vi "GetProbePlanCoordinates.vi"(8 "Use index as X coord":bool=TRUE, 9 "Probe Card Channels":i32=1) -> (0 "file path":string, 2 "OK?":bool, 3 "Array":T1(array[cluster]))   [LabVIEW 2018] (continued)
961\tX=-194.39\ty=30873.63 \nLabel=Strip\t962\tX=147.77\ty=30983.95 \nLabel=Strip\t963\tX=-206.37\ty=31022.23 \nLabel=Strip\t964\tX=135.75\ty=31132.68 \nLabel=Strip\t965\tX=-218.40\ty=31170.82 \nLabel=Strip\t966\tX=123.67\ty=31281.41 \nLabel=Strip\t967\tX=-230.49\ty=31319.41 \nLabel=Strip\t968\tX=111.54\ty=31430.13 \nLabel=Strip\t969\tX=-242.64\ty=31468.00 \nLabel=Strip\t970\tX=99.34\ty=31578.85 \nLabel=Strip\t971\tX=-254.85\ty=31616.58 \nLabel=Strip\t972\tX=87.09\ty=31727.56 \nLabel=Strip\t973\tX=-267.12\ty=31765.16 \nLabel=Strip\t974\tX=74.79\ty=31876.28 \nLabel=Strip\t975\tX=-279.44\ty=31913.74 \nLabel=Strip\t976\tX=62.42\ty=32024.98 \nLabel=Strip\t977\tX=-291.82\ty=32062.31 \nLabel=Strip\t978\tX=49.99\ty=32173.69 \nLabel=Strip\t979\tX=-304.26\ty=32210.88 \nLabel=Strip\t980\tX=37.51\ty=32322.39 \nLabel=Strip\t981\tX=-316.76\ty=32359.44 \nLabel=Strip\t982\tX=24.97\ty=32471.09 \nLabel=Strip\t983\tX=-329.31\ty=32508.01 \nLabel=Strip\t984\tX=12.38\ty=32619.78 \nLabel=Strip\t985\tX=-341.92\ty=32656.56 \nLabel=Strip\t986\tX=-0.28\ty=32768.47 \nLabel=Strip\t987\tX=-354.59\ty=32805.12 \nLabel=Strip\t988\tX=-12.99\ty=32917.16 \nLabel=Strip\t989\tX=-367.32\ty=32953.67 \nLabel=Strip\t990\tX=-25.76\ty=33065.85 \nLabel=Strip\t991\tX=-380.10\ty=33102.22 \nLabel=Strip\t992\tX=-38.59\ty=33214.53 \nLabel=Strip\t993\tX=-392.94\ty=33250.76 \nLabel=Strip\t994\tX=-51.47\ty=33363.20 \nLabel=Strip\t995\tX=-405.84\ty=33399.30 \nLabel=Strip\t996\tX=-64.41\ty=33511.88 \nLabel=Strip\t997\tX=-418.80\ty=33547.84 \nLabel=Strip\t998\tX=-77.42\ty=33660.55 \nLabel=Strip\t999\tX=-431.81\ty=33696.37 \nLabel=Strip\t1000\tX=-90.47\ty=33809.21 \nLabel=Strip\t1001\tX=-444.88\ty=33844.90 \nLabel=Strip\t1002\tX=-103.59\ty=33957.87 \nLabel=Strip\t1003\tX=-458.01\ty=33993.43 \nLabel=Strip\t1004\tX=-116.76\ty=34106.53 \nLabel=Strip\t1005\tX=-471.20\ty=34141.95 \nLabel=Strip\t1006\tX=-129.99\ty=34255.18 \nLabel=Strip\t1007\tX=-484.45\ty=34290.47 \nLabel=Strip\t1008\tX=-143.28\ty=34403.83 \nLabel=Strip\t1009\tX=-497.75\ty=34438.98 \nLabel=Strip\t1010\tX=-156.63\ty=34552.48 \nLabel=Strip\t1011\tX=-511.11\ty=34587.49 \nLabel=Strip\t1012\tX=-170.03\ty=34701.12 \nLabel=Strip\t1013\tX=-524.53\ty=34736.00 \nLabel=Strip\t1014\tX=-183.49\ty=34849.76 \nLabel=Strip\t1015\tX=-538.00\ty=34884.50 \nLabel=Strip\t1016\tX=-197.01\ty=34998.40 \nLabel=Strip\t1017\tX=-551.53\ty=35033.00 \nLabel=Strip\t1018\tX=-210.59\ty=35147.03 \nLabel=Strip\t1019\tX=-565.13\ty=35181.49 \nLabel=Strip\t1020\tX=-224.23\ty=35295.65 \nLabel=Strip\t1021\tX=-578.77\ty=35329.98 \nLabel=Strip\t1022\tX=-237.92\ty=35444.28 \nLabel=Strip\t1023\tX=-592.48\ty=35478.47 \nLabel=Strip\t1024\tX=-251.67\ty=35592.89 \nLabel=Strip\t1025\tX=-606.24\ty=35626.95 \nLabel=Strip\t1026\tX=-265.48\ty=35741.51 \nRegion=Segment\t3B\nLabel=Strip\t1\tX=16353.25\ty=-41866.46 \nLabel=Strip\t2\tX=16710.13\ty=-41818.03 \nLabel=Strip\t3\tX=16369.36\ty=-41712.09 \nLabel=Strip\t4\tX=16726.22\ty=-41663.53 \nLabel=Strip\t5\tX=16385.40\ty=-41557.71 \nLabel=Strip\t6\tX=16742.24\ty=-41509.01 \nLabel=Strip\t7\tX=16401.39\ty=-41403.33 \nLabel=Strip\t8\tX=16758.21\ty=-41354.49 \nLabel=Strip\t9\tX=16417.32\ty=-41248.94 \nLabel=Strip\t10\tX=16774.12\ty=-41199.96 \nLabel=Strip\t11\tX=16433.19\ty=-41094.54 \nLabel=Strip\t12\tX=16789.97\ty=-41045.43 \nLabel=Strip\t13\tX=16449.00\ty=-40940.14 \nLabel=Strip\t14\tX=16805.76\ty=-40890.88 \nLabel=Strip\t15\tX=16464.75\ty=-40785.73 \nLabel=Strip\t16\tX=16821.49\ty=-40736.33 \nLabel=Strip\t17\tX=16480.44\ty=-40631.31 \nLabel=Strip\t18\tX=16837.17\ty=-40581.78 \nLabel=Strip\t19\tX=16496.07\ty=-40476.88 \nLabel=Strip\t20\tX=16852.78\ty=-40427.21 \nLabel=Strip\t21\tX=16511.64\ty=-40322.44 \nLabel=Strip\t22\tX=16868.33\ty=-40272.64 \nLabel=Strip\t23\tX=16527.16\ty=-40168.00 \nLabel=Strip\t24\tX=16883.83\ty=-40118.06 \nLabel=Strip\t25\tX=16542.61\ty=-40013.55 \nLabel=Strip\t26\tX=16899.26\ty=-39963.47 \nLabel=Strip\t27\tX=16558.00\ty=-39859.10 \nLabel=Strip\t28\tX=16914.63\ty=-39808.88 \nLabel=Strip\t29\tX=16573.34\ty=-39704.63 \nLabel=Strip\t30\tX=16929.95\ty=-39654.27 \nLabel=Strip\t31\tX=16588.61\ty=-39550.16 \nLabel=Strip\t32\tX=16945.20\ty=-39499.66 \nLabel=Strip\t33\tX=16603.83\ty=-39395.69 \nLabel=Strip\t34\tX=16960.40\ty=-39345.05 \nLabel=Strip\t35\tX=16618.98\ty=-39241.20 \nLabel=Strip\t36\tX=16975.54\ty=-39190.43 \nLabel=Strip\t37\tX=16634.08\ty=-39086.71 \nLabel=Strip\t38\tX=16990.61\ty=-39035.80 \nLabel=Strip\t39\tX=16649.12\ty=-38932.21 \nLabel=Strip\t40\tX=17005.63\ty=-38881.16 \nLabel=Strip\t41\tX=16664.10\ty=-38777.70 \nLabel=Strip\t42\tX=17020.59\ty=-38726.51 \nLabel=Strip\t43\tX=16679.01\ty=-38623.19 \nLabel=Strip\t44\tX=17035.49\ty=-38571.86 \nLabel=Strip\t45\tX=16693.87\ty=-38468.67 \nLabel=Strip\t46\tX=17050.33\ty=-38417.20 \nLabel=Strip\t47\tX=16708.67\ty=-38314.14 \nLabel=Strip\t48\tX=17065.11\ty=-38262.54 \nLabel=Strip\t49\tX=16723.41\ty=-38159.61 \nLabel=Strip\t50\tX=17079.83\ty=-38107.86 \nLabel=Strip\t51\tX=16738.09\ty=-38005.07 \nLabel=Strip\t52\tX=17094.49\ty=-37953.18 \nLabel=Strip\t53\tX=16752.71\ty=-37850.52 \nLabel=Strip\t54\tX=17109.09\ty=-37798.50 \nLabel=Strip\t55\tX=16767.28\ty=-37695.96 \nLabel=Strip\t56\tX=17123.63\ty=-37643.80 \nLabel=Strip\t57\tX=16781.78\ty=-37541.40 \nLabel=Strip\t58\tX=17138.11\ty=-37489.10 \nLabel=Strip\t59\tX=16796.22\ty=-37386.83 \nLabel=Strip\t60\tX=17152.54\ty=-37334.40 \nLabel=Strip\t61\tX=16810.61\ty=-37232.26 \nLabel=Strip\t62\tX=17166.90\ty=-37179.68 \nLabel=Strip\t63\tX=16824.93\ty=-37077.67 \nLabel=Strip\t64\tX=17181.20\ty=-37024.96 \nLabel=Strip\t65\tX=16839.19\ty=-36923.08 \nLabel=Strip\t66\tX=17195.45\ty=-36870.23 \nLabel=Strip\t67\tX=16853.40\ty=-36768.49 \nLabel=Strip\t68\tX=17209.63\ty=-36715.50 \nLabel=Strip\t69\tX=16867.54\ty=-36613.89 \nLabel=Strip\t70\tX=17223.76\ty=-36560.76 \nLabel=Strip\t71\tX=16881.63\ty=-36459.28 \nLabel=Strip\t72\tX=17237.82\ty=-36406.01 \nLabel=Strip\t73\tX=16895.66\ty=-36304.66 \nLabel=Strip\t74\tX=17251.83\ty=-36251.26 \nLabel=Strip\t75\tX=16909.62\ty=-36150.04 \nLabel=Strip\t76\tX=17265.78\ty=-36096.49 \nLabel=Strip\t77\tX=16923.53\ty=-35995.41 \nLabel=Strip\t78\tX=17279.66\ty=-35941.73 \nLabel=Strip\t79\tX=16937.38\ty=-35840.77 \nLabel=Strip\t80\tX=17293.49\ty=-35786.95 \nLabel=Strip\t81\tX=16951.17\ty=-35686.13 \nLabel=Strip\t82\tX=17307.26\ty=-35632.17 \nLabel=Strip\t83\tX=16964.90\ty=-35531.48 \nLabel=Strip\t84\tX=17320.97\ty=-35477.38 \nLabel=Strip\t85\tX=16978.57\ty=-35376.82 \nLabel=Strip\t86\tX=17334.62\ty=-35322.59 \nLabel=Strip\t87\tX=16992.18\ty=-35222.16 \nLabel=Strip\t88\tX=17348.20\ty=-35167.79 \nLabel=Strip\t89\tX=17005.73\ty=-35067.49 \nLabel=Strip\t90\tX=17361.73\ty=-35012.98 \nLabel=Strip\t91\tX=17019.22\ty=-34912.81 \nLabel=Strip\t92\tX=17375.20\ty=-34858.17 \nLabel=Strip\t93\tX=17032.65\ty=-34758.13 \nLabel=Strip\t94\tX=17388.61\ty=-34703.35 \nLabel=Strip\t95\tX=17046.02\ty=-34603.44 \nLabel=Strip\t96\tX=17401.96\ty=-34548.52 \nLabel=Strip\t97\tX=17059.33\ty=-34448.75 \nLabel=Strip\t98\tX=17415.26\ty=-34393.68 \nLabel=Strip\t99\tX=17072.59\ty=-34294.04 \nLabel=Strip\t100\tX=17428.49\ty=-34238.85 \nLabel=Strip\t101\tX=17085.78\ty=-34139.34 \nLabel=Strip\t102\tX=17441.66\ty=-34084.00 \nLabel=Strip\t103\tX=17098.91\ty=-33984.62 \nLabel=Strip\t104\tX=17454.77\ty=-33929.15 \nLabel=Strip\t105\tX=17111.99\ty=-33829.90 \nLabel=Strip\t106\tX=17467.82\ty=-33774.29 \nLabel=Strip\t107\tX=17125.00\ty=-33675.17 \nLabel=Strip\t108\tX=17480.82\ty=-33619.42 \nLabel=Strip\t109\tX=17137.96\ty=-33520.44 \nLabel=Strip\t110\tX=17493.75\ty=-33464.55 \nLabel=Strip\t111\tX=17150.85\ty=-33365.70 \nLabel=Strip\t112\tX=17506.62\ty=-33309.67 \nLabel=Strip\t113\tX=17163.69\ty=-33210.95 \nLabel=Strip\t114\tX=17519.44\ty=-33154.79 \nLabel=Strip\t115\tX=17176.46\ty=-33056.20 \nLabel=Strip\t116\tX=17532.19\ty=-32999.90 \nLabel=Strip\t117\tX=17189.18\ty=-32901.44 \nLabel=Strip\t118\tX=17544.89\ty=-32845.00 \nLabel=Strip\t119\tX=17201.84\ty=-32746.68 \nLabel=Strip\t120\tX=17557.53\ty=-32690.10 \nLabel=Strip\t121\tX=17214.44\ty=-32591.91 \nLabel=Strip\t122\tX=17570.10\ty=-32535.19 \nLabel=Strip\t123\tX=17226.97\ty=-32437.13 \nLabel=Strip\t124\tX=17582.62\ty=-32380.28 \nLabel=Strip\t125\tX=17239.45\ty=-32282.35 \nLabel=Strip\t126\tX=17595.07\ty=-32225.35 \nLabel=Strip\t127\tX=17251.87\ty=-32127.65 \nLabel=Strip\t128\tX=17607.47\ty=-32070.43 \nLabel=Strip\t129\tX=17264.23\ty=-31972.76 \nLabel=Strip\t130\tX=17619.81\ty=-31915.49 \nLabel=Strip\t131\tX=17276.53\ty=-31817.96 \nLabel=Strip\t132\tX=17632.09\ty=-31760.55 \nLabel=Strip\t133\tX=17288.77\ty=-31663.15 \nLabel=Strip\t134\tX=17644.30\ty=-31605.61 \nLabel=Strip\t135\tX=17300.95\ty=-31508.34 \nLabel=Strip\t136\tX=17656.46\ty=-31450.66 \nLabel=Strip\t137\tX=17313.07\ty=-31353.52 \nLabel=Strip\t138\tX=17668.56\ty=-31295.70 \nLabel=Strip\t139\tX=17325.13\ty=-31198.70 \nLabel=Strip\t140\tX=17680.60\ty=-31140.74 \nLabel=Strip\t141\tX=17337.13\ty=-31043.86 \nLabel=Strip\t142\tX=17692.58\ty=-30985.77 \nLabel=Strip\t143\tX=17349.08\ty=-30889.03 \nLabel=Strip\t144\tX=17704.50\ty=-30830.79 \nLabel=Strip\t145\tX=17360.96\ty=-30734.18 \nLabel=Strip\t146\tX=17716.36\ty=-30675.81 \nLabel=Strip\t147\tX=17372.78\ty=-30579.33 \nLabel=Strip\t148\tX=17728.16\ty=-30520.82 \nLabel=Strip\t149\tX=17384.55\ty=-30424.48 \nLabel=Strip\t150\tX=17739.90\ty=-30365.83 \nLabel=Strip\t151\tX=17396.25\ty=-30269.62 \nLabel=Strip\t152\tX=17751.58\ty=-30210.83 \nLabel=Strip\t153\tX=17407.89\ty=-30114.75 \nLabel=Strip\t154\tX=17763.20\ty=-30055.83 \nLabel=Strip\t155\tX=17419.48\ty=-29959.88 \nLabel=Strip\t156\tX=17774.76\ty=-29900.82 \nLabel=Strip\t157\tX=17431.00\ty=-29805.00 \nLabel=Strip\t158\tX=17786.27\ty=-29745.80 \nLabel=Strip\t159\tX=17442.47\ty=-29650.12 \nLabel=Strip\t160\tX=17797.71\ty=-29590.78 \nLabel=Strip\t161\tX=17453.87\ty=-29495.23 \nLabel=Strip\t162\tX=17809.09\ty=-29435.75 \nLabel=Strip\t163\tX=17465.22\ty=-29340.33 \nLabel=Strip\t164\tX=17820.42\ty=-29280.72 \nLabel=Strip\t165\tX=17476.51\ty=-29185.43 \nLabel=Strip\t166\tX=17831.68\ty=-29125.68 \nLabel=Strip\t167\tX=17487.73\ty=-29030.53 \nLabel=Strip\t168\tX=17842.88\ty=-28970.64 \nLabel=Strip\t169\tX=17498.90\ty=-28875.61 \nLabel=Strip\t170\tX=17854.03\ty=-28815.59 \nLabel=Strip\t171\tX=17510.01\ty=-28720.70 \nLabel=Strip\t172\tX=17865.11\ty=-28660.53 \nLabel=Strip\t173\tX=17521.05\ty=-28565.77 \nLabel=Strip\t174\tX=17876.13\ty=-28505.47 \nLabel=Strip\t175\tX=17532.04\ty=-28410.84 \nLabel=Strip\t176\tX=17887.10\ty=-28350.41 \nLabel=Strip\t177\tX=17542.97\ty=-28255.91 \nLabel=Strip\t178\tX=17898.00\ty=-28195.33 \nLabel=Strip\t179\tX=17553.84\ty=-28100.97 \nLabel=Strip\t180\tX=17908.85\ty=-28040.25 \nLabel=Strip\t181\tX=17564.65\ty=-27946.03 \nLabel=Strip\t182\tX=17919.64\ty=-27885.17 \nLabel=Strip\t183\tX=17575.40\ty=-27791.07 \nLabel=Strip\t184\tX=17930.36\ty=-27730.08 \nLabel=Strip\t185\tX=17586.09\ty=-27636.12 \nLabel=Strip\t186\tX=17941.03\ty=-27574.99 \nLabel=Strip\t187\tX=17596.72\ty=-27481.16 \nLabel=Strip\t188\tX=17951.63\ty=-27419.89 \nLabel=Strip\t189\tX=17607.29\ty=-27326.19 \nLabel=Strip\t190\tX=17962.18\ty=-27264.79 \nLabel=Strip\t191\tX=17617.80\ty=-27171.22 \nLabel=Strip\t192\tX=17972.67\ty=-27109.68 \nLabel=Strip\t193\tX=17628.25\ty=-27016.24 \nLabel=Strip\t194\tX=17983.09\ty=-26954.56 \nLabel=Strip\t195\tX=17638.64\ty=-26861.26 \nLabel=Strip\t196\tX=17993.46\ty=-26799.44 \nLabel=Strip\t197\tX=17648.97\ty=-26706.27 \nLabel=Strip\t198\tX=18003.77\ty=-26644.31 \nLabel=Strip\t199\tX=17659.24\ty=-26551.27 \nLabel=Strip\t200\tX=18014.02\ty=-26489.18 \nLabel=Strip\t201\tX=17669.45\ty=-26396.28 \nLabel=Strip\t202\tX=18024.20\ty=-26334.05 \nLabel=Strip\t203\tX=17679.61\ty=-26241.27 \nLabel=Strip\t204\tX=18034.33\ty=-26178.90 \nLabel=Strip\t205\tX=17689.70\ty=-26086.26 \nLabel=Strip\t206\tX=18044.40\ty=-26023.76 \nLabel=Strip\t207\tX=17699.73\ty=-25931.25 \nLabel=Strip\t208\tX=18054.41\ty=-25868.60 \nLabel=Strip\t209\tX=17709.71\ty=-25776.23 \nLabel=Strip\t210\tX=18064.36\ty=-25713.45 \nLabel=Strip\t211\tX=17719.62\ty=-25621.20 \nLabel=Strip\t212\tX=18074.25\ty=-25558.28 \nLabel=Strip\t213\tX=17729.47\ty=-25466.17 \nLabel=Strip\t214\tX=18084.08\ty=-25403.12 \nLabel=Strip\t215\tX=17739.27\ty=-25311.14 \nLabel=Strip\t216\tX=18093.85\ty=-25247.94 \nLabel=Strip\t217\tX=17749.00\ty=-25156.10 \nLabel=Strip\t218\tX=18103.56\ty=-25092.77 \nLabel=Strip\t219\tX=17758.68\ty=-25001.05 \nLabel=Strip\t220\tX=18113.21\ty=-24937.58 \nLabel=Strip\t221\tX=17768.29\ty=-24846.00 \nLabel=Strip\t222\tX=18122.80\ty=-24782.40 \nLabel=Strip\t223\tX=17777.85\ty=-24690.95 \nLabel=Strip\t224\tX=18132.33\ty=-24627.20 \nLabel=Strip\t225\tX=17787.34\ty=-24535.89 \nLabel=Strip\t226\tX=18141.80\ty=-24472.01 \nLabel=Strip\t227\tX=17796.78\ty=-24380.82 \nLabel=Strip\t228\tX=18151.21\ty=-24316.80 \nLabel=Strip\t229\tX=17806.15\ty=-24225.75 \nLabel=Strip\t230\tX=18160.56\ty=-24161.59 \nLabel=Strip\t231\tX=17815.47\ty=-24070.68 \nLabel=Strip\t232\tX=18169.85\ty=-24006.38 \nLabel=Strip\t233\tX=17824.73\ty=-23915.60 \nLabel=Strip\t234\tX=18179.09\ty=-23851.17 \nLabel=Strip\t235\tX=17833.92\ty=-23760.51 \nLabel=Strip\t236\tX=18188.26\ty=-23695.94 \nLabel=Strip\t237\tX=17843.06\ty=-23605.42 \nLabel=Strip\t238\tX=18197.37\ty=-23540.72 \nLabel=Strip\t239\tX=17852.14\ty=-23450.33 \nLabel=Strip\t240\tX=18206.42\ty=-23385.48 \nLabel=Strip\t241\tX=17861.15\ty=-23295.23 \nLabel=Strip\t242\tX=18215.41\ty=-23230.25 \nLabel=Strip\t243\tX=17870.11\ty=-23140.12 \nLabel=Strip\t244\tX=18224.35\ty=-23075.01 \nLabel=Strip\t245\tX=17879.01\ty=-22985.02 \nLabel=Strip\t246\tX=18233.22\ty=-22919.76 \nLabel=Strip\t247\tX=17887.85\ty=-22829.90 \nLabel=Strip\t248\tX=18242.05\ty=-22764.05 \nLabel=Strip\t249\tX=17896.63\ty=-22674.78 \nLabel=Strip\t250\tX=18250.79\ty=-22609.25 \nLabel=Strip\t251\tX=17905.34\ty=-22519.66 \nLabel=Strip\t252\tX=18259.48\ty=-22453.99 \nLabel=Strip\t253\tX=17914.00\ty=-22364.53 \nLabel=Strip\t254\tX=18268.11\ty=-22298.73 \nLabel=Strip\t255\tX=17922.60\ty=-22209.40 \nLabel=Strip\t256\tX=18276.69\ty=-22143.46 \nLabel=Strip\t257\tX=17931.14\ty=-22054.27 \nLabel=Strip\t258\tX=18285.20\ty=-21988.18 \nLabel=Strip\t259\tX=17939.62\ty=-21899.12 \nLabel=Strip\t260\tX=18293.65\ty=-21832.91 \nLabel=Strip\t261\tX=17948.04\ty=-21743.98 \nLabel=Strip\t262\tX=18302.05\ty=-21677.62 \nLabel=Strip\t263\tX=17956.40\ty=-21588.83 \nLabel=Strip\t264\tX=18310.38\ty=-21522.33 \nLabel=Strip\t265\tX=17964.70\ty=-21433.67 \nLabel=Strip\t266\tX=18318.66\ty=-21367.04 \nLabel=Strip\t267\tX=17972.94\ty=-21278.51 \nLabel=Strip\t268\tX=18326.87\ty=-21211.75 \nLabel=Strip\t269\tX=17981.12\ty=-21123.35 \nLabel=Strip\t270\tX=18335.03\ty=-21056.44 \nLabel=Strip\t271\tX=17989.24\ty=-20968.18 \nLabel=Strip\t272\tX=18343.12\ty=-20901.14 \nLabel=Strip\t273\tX=17997.30\ty=-20813.01 \nLabel=Strip\t274\tX=18351.16\ty=-20745.83 \nLabel=Strip\t275\tX=18005.30\ty=-20657.83 \nLabel=Strip\t276\tX=18359.13\ty=-20590.51 \nLabel=Strip\t277\tX=18013.24\ty=-20502.65 \nLabel=Strip\t278\tX=18367.05\ty=-20435.20 \nLabel=Strip\t279\tX=18021.13\ty=-20347.46 \nLabel=Strip\t280\tX=18374.90\ty=-20279.87 \nLabel=Strip\t281\tX=18028.95\ty=-20192.27 \nLabel=Strip\t282\tX=18382.70\ty=-20124.55 \nLabel=Strip\t283\tX=18036.71\ty=-20037.08 \nLabel=Strip\t284\tX=18390.43\ty=-19969.21 \nLabel=Strip\t285\tX=18044.41\ty=-19881.88 \nLabel=Strip\t286\tX=18398.11\ty=-19813.88 \nLabel=Strip\t287\tX=18052.05\ty=-19726.68 \nLabel=Strip\t288\tX=18405.72\ty=-19658.54 \nLabel=Strip\t289\tX=18059.64\ty=-19571.47 \nLabel=Strip\t290\tX=18413.28\ty=-19503.19 \nLabel=Strip\t291\tX=18067.16\ty=-19416.26 \nLabel=Strip\t292\tX=18420.78\ty=-19347.84 \nLabel=Strip\t293\tX=18074.62\ty=-19261.04 \nLabel=Strip\t294\tX=18428.21\ty=-19192.49 \nLabel=Strip\t295\tX=18082.02\ty=-19105.82 \nLabel=Strip\t296\tX=18435.59\ty=-19037.13 \nLabel=Strip\t297\tX=18089.37\ty=-18950.60 \nLabel=Strip\t298\tX=18442.91\ty=-18881.77 \nLabel=Strip\t299\tX=18096.65\ty=-18795.37 \nLabel=Strip\t300\tX=18450.16\ty=-18726.41 \nLabel=Strip\t301\tX=18103.87\ty=-18640.14 \nLabel=Strip\t302\tX=18457.36\ty=-18571.04 \nLabel=Strip\t303\tX=18111.04\ty=-18484.90 \nLabel=Strip\t304\tX=18464.50\ty=-18415.66 \nLabel=Strip\t305\tX=18118.14\ty=-18329.66 \nLabel=Strip\t306\tX=18471.57\ty=-18260.29 \nLabel=Strip\t307\tX=18125.18\ty=-18174.42 \nLabel=Strip\t308\tX=18478.59\ty=-18104.90 \nLabel=Strip\t309\tX=18132.17\ty=-18019.17 \nLabel=Strip\t310\tX=18485.55\ty=-17949.52 \nLabel=Strip\t311\tX=18139.09\ty=-17863.91 \nLabel=Strip\t312\tX=18492.44\ty=-17794.13 \nLabel=Strip\t313\tX=18145.96\ty=-17708.66 \nLabel=Strip\t314\tX=18499.28\ty=-17638.73 \nLabel=Strip\t315\tX=18152.76\ty=-17553.40 \nLabel=Strip\t316\tX=18506.06\ty=-17483.34 \nLabel=Strip\t317\tX=18159.50\ty=-17398.13 \nLabel=Strip\t318\tX=18512.78\ty=-17327.94 \nLabel=Strip\t319\tX=18166.19\ty=-17242.86 \nLabel=Strip\t320\tX=18519.43\ty=-17172.53 \nLabel=Strip\t321\tX=18172.81\ty=-17087.59 \nLabel=Strip\t322\tX=18526.03\ty=-17017.12 \nLabel=Strip\t323\tX=18179.38\ty=-16932.32 \nLabel=Strip\t324\tX=18532.57\ty=-16861.71 \nLabel=Strip\t325\tX=18185.88\ty=-16777.04 \nLabel=Strip\t326\tX=18539.05\ty=-16706.29 \nLabel=Strip\t327\tX=18192.33\ty=-16621.75 \nLabel=Strip\t328\tX=18545.46\ty=-16550.87 \nLabel=Strip\t329\tX=18198.71\ty=-16466.45 \nLabel=Strip\t330\tX=18551.82\ty=-16395.45 \nLabel=Strip\t331\tX=18205.04\ty=-16311.17 \nLabel=Strip\t332\tX=18558.12\ty=-16240.02 \nLabel=Strip\t333\tX=18211.30\ty=-16155.88 \nLabel=Strip\t334\tX=18564.36\ty=-16084.59 \nLabel=Strip\t335\tX=18217.51\ty=-16000.58 \nLabel=Strip\t336\tX=18570.54\ty=-15929.15 \nLabel=Strip\t337\tX=18223.66\ty=-15845.28 \nLabel=Strip\t338\tX=18576.65\ty=-15773.71 \nLabel=Strip\t339\tX=18229.74\ty=-15689.97 \nLabel=Strip\t340\tX=18582.71\ty=-15618.27 \nLabel=Strip\t341\tX=18235.77\ty=-15534.66 \nLabel=Strip\t342\tX=18588.71\ty=-15462.82 \nLabel=Strip\t343\tX=18241.73\ty=-15379.35 \nLabel=Strip\t344\tX=18594.65\ty=-15307.37 \nLabel=Strip\t345\tX=18247.64\ty=-15224.03 \nLabel=Strip\t346\tX=18600.53\ty=-15151.92 \nLabel=Strip\t347\tX=18253.49\ty=-15068.71 \nLabel=Strip\t348\tX=18606.35\ty=-14996.46 \nLabel=Strip\t349\tX=18259.27\ty=-14913.39 \nLabel=Strip\t350\tX=18612.10\ty=-14841.00 \nLabel=Strip\t351\tX=18265.00\ty=-14758.06 \nLabel=Strip\t352\tX=18617.80\ty=-14685.53 \nLabel=Strip\t353\tX=18270.67\ty=-14602.73 \nLabel=Strip\t354\tX=18623.44\ty=-14530.07 \nLabel=Strip\t355\tX=18276.27\ty=-14447.40 \nLabel=Strip\t356\tX=18629.02\ty=-14374.60 \nLabel=Strip\t357\tX=18281.82\ty=-14292.06 \nLabel=Strip\t358\tX=18634.54\ty=-14219.12 \nLabel=Strip\t359\tX=18287.31\ty=-14136.72 \nLabel=Strip\t360\tX=18640.00\ty=-14063.64 \nLabel=Strip\t361\tX=18292.73\ty=-13981.37 \nLabel=Strip\t362\tX=18645.40\ty=-13908.16 \nLabel=Strip\t363\tX=18298.10\ty=-13826.02 \nLabel=Strip\t364\tX=18650.73\ty=-13752.68 \nLabel=Strip\t365\tX=18303.41\ty=-13670.67 \nLabel=Strip\t366\tX=18656.01\ty=-13597.19 \nLabel=Strip\t367\tX=18308.65\ty=-13515.32 \nLabel=Strip\t368\tX=18661.23\ty=-13441.70 \nLabel=Strip\t369\tX=18313.84\ty=-13359.96 \nLabel=Strip\t370\tX=18666.39\ty=-13286.20 \nLabel=Strip\t371\tX=18318.97\ty=-13204.60 \nLabel=Strip\t372\tX=18671.49\ty=-13130.70 \nLabel=Strip\t373\tX=18324.04\ty=-13049.23 \nLabel=Strip\t374\tX=18676.53\ty=-12975.20 \nLabel=Strip\t375\tX=18329.04\ty=-12893.86 \nLabel=Strip\t376\tX=18681.51\ty=-12819.70 \nLabel=Strip\t377\tX=18333.99\ty=-12738.49 \nLabel=Strip\t378\tX=18686.43\ty=-12664.19 \nLabel=Strip\t379\tX=18338.88\ty=-12583.12 \nLabel=Strip\t380\tX=18691.28\ty=-12508.68 \nLabel=Strip\t381\tX=18343.71\ty=-12427.74 \nLabel=Strip\t382\tX=18696.08\ty=-12353.16 \nLabel=Strip\t383\tX=18348.47\ty=-12272.36 \nLabel=Strip\t384\tX=18700.82\ty=-12197.64 \nLabel=Strip\t385\tX=18353.18\ty=-12116.98 \nLabel=Strip\t386\tX=18705.50\ty=-12042.12 \nLabel=Strip\t387\tX=18357.83\ty=-11961.59 \nLabel=Strip\t388\tX=18710.12\ty=-11886.60 \nLabel=Strip\t389\tX=18362.42\ty=-11806.20 \nLabel=Strip\t390\tX=18714.68\ty=-11731.07 \nLabel=Strip\t391\tX=18366.94\ty=-11650.80 \nLabel=Strip\t392\tX=18719.18\ty=-11575.54 \nLabel=Strip\t393\tX=18371.41\ty=-11495.41 \nLabel=Strip\t394\tX=18723.62\ty=-11420.01 \nLabel=Strip\t395\tX=18375.82\ty=-11340.01 \nLabel=Strip\t396\tX=18728.00\ty=-11264.47 \nLabel=Strip\t397\tX=18380.17\ty=-11184.61 \nLabel=Strip\t398\tX=18732.31\ty=-11108.93 \nLabel=Strip\t399\tX=18384.46\ty=-11029.20 \nLabel=Strip\t400\tX=18736.57\ty=-10953.39 \nLabel=Strip\t401\tX=18388.68\ty=-10873.79 \nLabel=Strip\t402\tX=18740.77\ty=-10797.85 \nLabel=Strip\t403\tX=18392.85\ty=-10718.38 \nLabel=Strip\t404\tX=18744.91\ty=-10642.30 \nLabel=Strip\t405\tX=18397.03\ty=-10545.69 \nLabel=Strip\t406\tX=18749.04\ty=-10472.72 \nLabel=Strip\t407\tX=18401.05\ty=-10397.30 \nLabel=Strip\t408\tX=18753.03\ty=-10324.33 \nLabel=Strip\t409\tX=18405.01\ty=-10248.90 \nLabel=Strip\t410\tX=18756.97\ty=-10175.93 \nLabel=Strip\t411\tX=18408.91\ty=-10100.50 \nLabel=Strip\t412\tX=18760.84\ty=-10027.53 \nLabel=Strip\t413\tX=18412.76\ty=-9952.10 \nLabel=Strip\t414\tX=18764.66\ty=-9879.13 \nLabel=Strip\t415\tX=18416.55\ty=-9803.70 \nLabel=Strip\t416\tX=18768.48\ty=-9708.95 \nLabel=Strip\t417\tX=18420.35\ty=-9630.42 \nLabel=Strip\t418\tX=18772.20\ty=-9553.39 \nLabel=Strip\t419\tX=18424.04\ty=-9474.99 \nLabel=Strip\t420\tX=18775.86\ty=-9397.82 \nLabel=Strip\t421\tX=18427.67\ty=-9319.55 \nLabel=Strip\t422\tX=18779.46\ty=-9242.24 \nLabel=Strip\t423\tX=18431.23\ty=-9164.11 \nLabel=Strip\t424\tX=18783.00\ty=-9086.67 \nLabel=Strip\t425\tX=18434.74\ty=-9008.67 \nLabel=Strip\t426\tX=18786.48\ty=-8931.09 \nLabel=Strip\t427\tX=18438.19\ty=-8853.23 \nLabel=Strip\t428\tX=18789.89\ty=-8775.51 \nLabel=Strip\t429\tX=18441.58\ty=-8697.78 \nLabel=Strip\t430\tX=18793.25\ty=-8619.92 \nLabel=Strip\t431\tX=18444.91\ty=-8542.33 \nLabel=Strip\t432\tX=18796.55\ty=-8464.34 \nLabel=Strip\t433\tX=18448.18\ty=-8386.88 \nLabel=Strip\t434\tX=18799.79\ty=-8308.75 \nLabel=Strip\t435\tX=18451.39\ty=-8231.42 \nLabel=Strip\t436\tX=18802.97\ty=-8153.16 \nLabel=Strip\t437\tX=18454.53\ty=-8075.97 \nLabel=Strip\t438\tX=18806.08\ty=-7997.56 \nLabel=Strip\t439\tX=18457.62\ty=-7920.51 \nLabel=Strip\t440\tX=18809.14\ty=-7841.97 \nLabel=Strip\t441\tX=18460.65\ty=-7765.04 \nLabel=Strip\t442\tX=18812.14\ty=-7686.37 \nLabel=Strip\t443\tX=18463.62\ty=-7609.58 \nLabel=Strip\t444\tX=18815.08\ty=-7530.77 \nLabel=Strip\t445\tX=18466.53\ty=-7454.11 \nLabel=Strip\t446\tX=18817.96\ty=-7375.16 \nLabel=Strip\t447\tX=18469.38\ty=-7298.64 \nLabel=Strip\t448\tX=18820.77\ty=-7219.56 \nLabel=Strip\t449\tX=18472.16\ty=-7143.17 \nLabel=Strip\t450\tX=18823.53\ty=-7063.95 \nLabel=Strip\t451\tX=18474.89\ty=-6987.70 \nLabel=Strip\t452\tX=18826.23\ty=-6908.34 \nLabel=Strip\t453\tX=18477.56\ty=-6832.22 \nLabel=Strip\t454\tX=18828.87\ty=-6752.73 \nLabel=Strip\t455\tX=18480.17\ty=-6676.74 \nLabel=Strip\t456\tX=18831.45\ty=-6597.11 \nLabel=Strip\t457\tX=18482.72\ty=-6521.26 \nLabel=Strip\t458\tX=18833.96\ty=-6441.49 \nLabel=Strip\t459\tX=18485.21\ty=-6365.77 \nLabel=Strip\t460\tX=18836.42\ty=-6285.87 \nLabel=Strip\t461\tX=18487.63\ty=-6210.29 \nLabel=Strip\t462\tX=18838.82\ty=-6130.25 \nLabel=Strip\t463\tX=18490.00\ty=-6054.80 \nLabel=Strip\t464\tX=18841.16\ty=-5974.62 \nLabel=Strip\t465\tX=18492.31\ty=-5899.31 \nLabel=Strip\t466\tX=18843.43\ty=-5819.00 \nLabel=Strip\t467\tX=18494.56\ty=-5743.82 \nLabel=Strip\t468\tX=18845.65\ty=-5663.37 \nLabel=Strip\t469\tX=18496.75\ty=-5588.32 \nLabel=Strip\t470\tX=18847.81\ty=-5507.74 \nLabel=Strip\t471\tX=18498.88\ty=-5432.82 \nLabel=Strip\t472\tX=18849.90\ty=-5352.10 \nLabel=Strip\t473\tX=18500.94\ty=-5277.33 \nLabel=Strip\t474\tX=18851.94\ty=-5196.47 \nLabel=Strip\t475\tX=18502.95\ty=-5121.82 \nLabel=Strip\t476\tX=18853.92\ty=-5040.83 \nLabel=Strip\t477\tX=18504.90\ty=-4966.32 \nLabel=Strip\t478\tX=18855.83\ty=-4885.19 \nLabel=Strip\t479\tX=18506.79\ty=-4810.82 \nLabel=Strip\t480\tX=18857.69\ty=-4729.55 \nLabel=Strip\t481\tX=18508.62\ty=-4655.31 \nLabel=Strip\t482\tX=18859.49\ty=-4573.91 \nLabel=Strip\t483\tX=18510.38\ty=-4499.80 \nLabel=Strip\t484\tX=18861.22\ty=-4418.26 \nLabel=Strip\t485\tX=18512.09\ty=-4344.29 \nLabel=Strip\t486\tX=18862.90\ty=-4262.62 \nLabel=Strip\t487\tX=18513.74\ty=-4188.77 \nLabel=Strip\t488\tX=18864.52\ty=-4106.97 \nLabel=Strip\t489\tX=18515.33\ty=-4033.26 \nLabel=Strip\t490\tX=18866.07\ty=-3951.31 \nLabel=Strip\t491\tX=18516.85\ty=-3877.74 \nLabel=Strip\t492\tX=18867.57\ty=-3795.66 \nLabel=Strip\t493\tX=18518.32\ty=-3722.22 \nLabel=Strip\t494\tX=18869.00\ty=-3640.01 \nLabel=Strip\t495\tX=18519.73\ty=-3566.70 \nLabel=Strip\t496\tX=18870.38\ty=-3484.35 \nLabel=Strip\t497\tX=18521.08\ty=-3411.18 \nLabel=Strip\t498\tX=18871.70\ty=-3328.69 \nLabel=Strip\t499\tX=18522.37\ty=-3255.66 \nLabel=Strip\t500\tX=18872.95\ty=-3173.03 \nLabel=Strip\t501\tX=18523.59\ty=-3100.13 \nLabel=Strip\t502\tX=18874.15\ty=-3017.37 \nLabel=Strip\t503\tX=18524.76\ty=-2944.60 \nLabel=Strip\t504\tX=18875.28\ty=-2861.70 \nLabel=Strip\t505\tX=18525.87\ty=-2789.07 \nLabel=Strip\t506\tX=18876.36\ty=-2706.02 \nLabel=Strip\t507\tX=18526.91\ty=-2633.54 \nLabel=Strip\t508\tX=18877.37\ty=-2550.37 \nLabel=Strip\t509\tX=18527.90\ty=-2478.01 \nLabel=Strip\t510\tX=18878.33\ty=-2394.70 \nLabel=Strip\t511\tX=18528.83\ty=-2322.47 \nLabel=Strip\t512\tX=18879.22\ty=-2239.03 \nLabel=Strip\t513\tX=18529.70\ty=-2166.93 \nLabel=Strip\t514\tX=18880.06\ty=-2083.36 \nLabel=Strip\t515\tX=18530.50\ty=-2011.40 \nLabel=Strip\t516\tX=18880.83\ty=-1927.68 \nLabel=Strip\t517\tX=18531.25\ty=-1855.86 \nLabel=Strip\t518\tX=18881.55\ty=-1772.01 \nLabel=Strip\t519\tX=18531.94\ty=-1700.31 \nLabel=Strip\t520\tX=18882.20\ty=-1616.33 \nLabel=Strip\t521\tX=18532.56\ty=-1544.77 \nLabel=Strip\t522\tX=18882.80\ty=-1460.65 \nLabel=Strip\t523\tX=18533.13\ty=-1389.23 \nLabel=Strip\t524\tX=18883.33\ty=-1304.97 \nLabel=Strip\t525\tX=18533.64\ty=-1233.68 \nLabel=Strip\t526\tX=18883.81\ty=-1149.29 \nLabel=Strip\t527\tX=18534.08\ty=-1078.13 \nLabel=Strip\t528\tX=18884.22\ty=-993.61 \nLabel=Strip\t529\tX=18534.47\ty=-922.58 \nLabel=Strip\t530\tX=18884.57\ty=-837.92 \nLabel=Strip\t531\tX=18534.80\ty=-767.03 \nLabel=Strip\t532\tX=18884.87\ty=-682.23 \nLabel=Strip\t533\tX=18535.06\ty=-611.48 \nLabel=Strip\t534\tX=18885.10\ty=-526.55 \nLabel=Strip\t535\tX=18535.27\ty=-455.93 \nLabel=Strip\t536\tX=18885.27\ty=-370.86 \nLabel=Strip\t537\tX=18535.42\ty=-300.37 \nLabel=Strip\t538\tX=18885.39\ty=-215.17 \nLabel=Strip\t539\tX=18535.50\ty=-144.82 \nLabel=Strip\t540\tX=18885.44\ty=-59.47 \nLabel=Strip\t541\tX=18535.53\ty=10.74 \nLabel=Strip\t542\tX=18885.43\ty=96.22 \nLabel=Strip\t543\tX=18535.49\ty=166.30 \nLabel=Strip\t544\tX=18885.37\ty=251.91 \nLabel=Strip\t545\tX=18535.40\ty=321.86 \nLabel=Strip\t546\tX=18885.24\ty=407.61 \nLabel=Strip\t547\tX=18535.25\ty=477.42 \nLabel=Strip\t548\tX=18885.05\ty=563.31 \nLabel=Strip\t549\tX=18535.03\ty=632.98 \nLabel=Strip\t550\tX=18884.80\ty=719.00 \nLabel=Strip\t551\tX=18534.76\ty=788.54 \nLabel=Strip\t552\tX=18884.50\ty=874.70 \nLabel=Strip\t553\tX=18534.42\ty=944.11 \nLabel=Strip\t554\tX=18884.13\ty=1030.40 \nLabel=Strip\t555\tX=18534.03\ty=1099.68 \nLabel=Strip\t556\tX=18883.70\ty=1186.10 \nLabel=Strip\t557\tX=18533.57\ty=1255.24 \nLabel=Strip\t558\tX=18883.21\ty=1341.81 \nLabel=Strip\t559\tX=18533.06\ty=1410.81 \nLabel=Strip\t560\tX=18882.66\ty=1497.51 \nLabel=Strip\t561\tX=18532.48\ty=1566.38 \nLabel=Strip\t562\tX=18882.05\ty=1653.22 \nLabel=Strip\t563\tX=18531.85\ty=1721.95 \nLabel=Strip\t564\tX=18881.39\ty=1808.92 \nLabel=Strip\t565\tX=18531.15\ty=1877.52 \nLabel=Strip\t566\tX=18880.66\ty=1964.63 \nLabel=Strip\t567\tX=18530.40\ty=2033.09 \nLabel=Strip\t568\tX=18879.87\ty=2120.34 \nLabel=Strip\t569\tX=18529.58\ty=2188.67 \nLabel=Strip\t570\tX=18879.02\ty=2276.05 \nLabel=Strip\t571\tX=18528.71\ty=2344.24 \nLabel=Strip\t572\tX=18878.11\ty=2431.76 \nLabel=Strip\t573\tX=18527.77\ty=2499.82 \nLabel=Strip\t574\tX=18877.14\ty=2587.47 \nLabel=Strip\t575\tX=18526.77\ty=2655.39 \nLabel=Strip\t576\tX=18876.11\ty=2743.18 \nLabel=Strip\t577\tX=18525.72\ty=2810.97 \nLabel=Strip\t578\tX=18875.02\ty=2898.89 \nLabel=Strip\t579\tX=18524.60\ty=2966.55 \nLabel=Strip\t580\tX=18873.87\ty=3054.61 \nLabel=Strip\t581\tX=18523.43\ty=3122.13 \nLabel=Strip\t582\tX=18872.66\ty=3210.32 \nLabel=Strip\t583\tX=18522.19\ty=3277.71 \nLabel=Strip\t584\tX=18871.39\ty=3366.04 \nLabel=Strip\t585\tX=18520.89\ty=3433.29 \nLabel=Strip\t586\tX=18870.06\ty=3521.75 \nLabel=Strip\t587\tX=18519.54\ty=3588.87 \nLabel=Strip\t588\tX=18868.67\ty=3677.47 \nLabel=Strip\t589\tX=18518.12\ty=3744.45 \nLabel=Strip\t590\tX=18867.22\ty=3833.19 \nLabel=Strip\t591\tX=18516.64\ty=3900.04 \nLabel=Strip\t592\tX=18865.71\ty=3988.91 \nLabel=Strip\t593\tX=18515.11\ty=4055.62 \nLabel=Strip\t594\tX=18864.14\ty=4144.63 \nLabel=Strip\t595\tX=18513.51\ty=4211.20 \nLabel=Strip\t596\tX=18862.50\ty=4300.34 \nLabel=Strip\t597\tX=18511.85\ty=4366.79 \nLabel=Strip\t598\tX=18860.81\ty=4456.07 \nLabel=Strip\t599\tX=18510.14\ty=4522.38 \nLabel=Strip\t600\tX=18859.06\ty=4611.79 \nLabel=Strip\t601\tX=18508.36\ty=4677.96 \nLabel=Strip\t602\tX=18857.25\ty=4767.51 \nLabel=Strip\t603\tX=18506.52\ty=4833.55 \nLabel=Strip\t604\tX=18855.38\ty=4923.23 \nLabel=Strip\t605\tX=18504.62\ty=4989.14 \nLabel=Strip\t606\tX=18853.45\ty=5078.95 \nLabel=Strip\t607\tX=18502.67\ty=5144.73 \nLabel=Strip\t608\tX=18851.45\ty=5234.68 \nLabel=Strip\t609\tX=18500.65\ty=5300.31 \nLabel=Strip\t610\tX=18849.40\ty=5390.40 \nLabel=Strip\t611\tX=18498.57\ty=5455.90 \nLabel=Strip\t612\tX=18847.29\ty=5546.13 \nLabel=Strip\t613\tX=18496.43\ty=5611.49 \nLabel=Strip\t614\tX=18845.11\ty=5701.85 \nLabel=Strip\t615\tX=18494.23\ty=5767.08 \nLabel=Strip\t616\tX=18842.88\ty=5857.58 \nLabel=Strip\t617\tX=18491.97\ty=5922.67 \nLabel=Strip\t618\tX=18840.59\ty=6013.30 \nLabel=Strip\t619\tX=18489.66\ty=6078.26 \nLabel=Strip\t620\tX=18838.23\ty=6169.03 \nLabel=Strip\t621\tX=18487.28\ty=6233.86 \nLabel=Strip\t622\tX=18835.82\ty=6324.76 \nLabel=Strip\t623\tX=18484.84\ty=6389.45 \nLabel=Strip\t624\tX=18833.35\ty=6480.48 \nLabel=Strip\t625\tX=18482.34\ty=6545.04 \nLabel=Strip\t626\tX=18830.81\ty=6636.21 \nLabel=Strip\t627\tX=18479.78\ty=6700.63 \nLabel=Strip\t628\tX=18828.22\ty=6791.94 \nLabel=Strip\t629\tX=18477.16\ty=6856.23 \nLabel=Strip\t630\tX=18825.56\ty=6947.67 \nLabel=Strip\t631\tX=18474.48\ty=7011.82 \nLabel=Strip\t632\tX=18822.85\ty=7103.40 \nLabel=Strip\t633\tX=18471.74\ty=7167.41 \nLabel=Strip\t634\tX=18820.07\ty=7259.12 \nLabel=Strip\t635\tX=18468.94\ty=7323.01 \nLabel=Strip\t636\tX=18817.24\ty=7414.85 \nLabel=Strip\t637\tX=18466.08\ty=7478.60 \nLabel=Strip\t638\tX=18814.34\ty=7570.58 \nLabel=Strip\t639\tX=18463.16\ty=7634.19 \nLabel=Strip\t640\tX=18811.39\ty=7726.31 \nLabel=Strip\t641\tX=18460.18\ty=7789.79 \nLabel=Strip\t642\tX=18808.37\ty=7882.04 \nLabel=Strip\t643\tX=18457.14\ty=7945.38 \nLabel=Strip\t644\tX=18805.29\ty=8037.77 \nLabel=Strip\t645\tX=18454.04\ty=8100.98 \nLabel=Strip\t646\tX=18802.16\ty=8193.50 \nLabel=Strip\t647\tX=18450.88\ty=8256.57 \nLabel=Strip\t648\tX=18798.96\ty=8349.23 \nLabel=Strip\t649\tX=18447.66\ty=8412.17 \nLabel=Strip\t650\tX=18795.70\ty=8504.96 \nLabel=Strip\t651\tX=18444.38\ty=8567.76 \nLabel=Strip\t652\tX=18792.39\ty=8660.69 \nLabel=Strip\t653\tX=18441.04\ty=8723.36 \nLabel=Strip\t654\tX=18789.01\ty=8816.42 \nLabel=Strip\t655\tX=18437.64\ty=8878.95 \nLabel=Strip\t656\tX=18785.57\ty=8972.15 \nLabel=Strip\t657\tX=18434.17\ty=9034.54 \nLabel=Strip\t658\tX=18782.08\ty=9127.88 \nLabel=Strip\t659\tX=18430.65\ty=9190.14 \nLabel=Strip\t660\tX=18778.52\ty=9283.61 \nLabel=Strip\t661\tX=18427.07\ty=9345.73 \nLabel=Strip\t662\tX=18774.90\ty=9439.34 \nLabel=Strip\t663\tX=18423.43\ty=9501.33 \nLabel=Strip\t664\tX=18771.22\ty=9595.07 \nLabel=Strip\t665\tX=18419.73\ty=9656.92 \nLabel=Strip\t666\tX=18767.48\ty=9750.80 \nLabel=Strip\t667\tX=18415.96\ty=9812.52 \nLabel=Strip\t668\tX=18763.68\ty=9906.52 \nLabel=Strip\t669\tX=18412.14\ty=9968.11 \nLabel=Strip\t670\tX=18759.83\ty=10062.25 \nLabel=Strip\t671\tX=18408.26\ty=10123.71 \nLabel=Strip\t672\tX=18755.91\ty=10217.98 \nLabel=Strip\t673\tX=18404.32\ty=10279.30 \nLabel=Strip\t674\tX=18751.93\ty=10373.71 \nLabel=Strip\t675\tX=18400.31\ty=10434.89 \nLabel=Strip\t676\tX=18747.89\ty=10529.44 \nLabel=Strip\t677\tX=18396.25\ty=10590.49 \nLabel=Strip\t678\tX=18743.79\ty=10685.17 \nLabel=Strip\t679\tX=18392.13\ty=10746.08 \nLabel=Strip\t680\tX=18739.63\ty=10840.90 \nLabel=Strip\t681\tX=18387.94\ty=10901.67 \nLabel=Strip\t682\tX=18735.41\ty=10996.62 \nLabel=Strip\t683\tX=18383.70\ty=11057.26 \nLabel=Strip\t684\tX=18731.13\ty=11152.35 \nLabel=Strip\t685\tX=18379.40\ty=11212.86 \nLabel=Strip\t686\tX=18726.79\ty=11308.08 \nLabel=Strip\t687\tX=18375.03\ty=11368.45 \nLabel=Strip\t688\tX=18722.39\ty=11463.80 \nLabel=Strip\t689\tX=18370.61\ty=11524.04 \nLabel=Strip\t690\tX=18717.92\ty=11619.53 \nLabel=Strip\t691\tX=18366.12\ty=11679.63 \nLabel=Strip\t692\tX=18713.40\ty=11775.25 \nLabel=Strip\t693\tX=18361.58\ty=11835.22 \nLabel=Strip\t694\tX=18708.82\ty=11930.98 \nLabel=Strip\t695\tX=18356.97\ty=11990.81 \nLabel=Strip\t696\tX=18704.18\ty=12086.70 \nLabel=Strip\t697\tX=18352.31\ty=12146.40 \nLabel=Strip\t698\tX=18699.48\ty=12242.43 \nLabel=Strip\t699\tX=18347.58\ty=12301.99 \nLabel=Strip\t700\tX=18694.72\ty=12398.15 \nLabel=Strip\t701\tX=18342.80\ty=12457.58 \nLabel=Strip\t702\tX=18689.89\ty=12553.88 \nLabel=Strip\t703\tX=18337.95\ty=12613.16 \nLabel=Strip\t704\tX=18685.01\ty=12709.60 \nLabel=Strip\t705\tX=18333.05\ty=12768.75 \nLabel=Strip\t706\tX=18680.07\ty=12865.32 \nLabel=Strip\t707\tX=18328.08\ty=12924.34 \nLabel=Strip\t708\tX=18675.06\ty=13021.04 \nLabel=Strip\t709\tX=18323.05\ty=13079.92 \nLabel=Strip\t710\tX=18670.00\ty=13176.76 \nLabel=Strip\t711\tX=18317.97\ty=13235.51 \nLabel=Strip\t712\tX=18664.88\ty=13332.48 \nLabel=Strip\t713\tX=18312.82\ty=13391.09 \nLabel=Strip\t714\tX=18659.69\ty=13488.20 \nLabel=Strip\t715\tX=18307.62\ty=13546.68 \nLabel=Strip\t716\tX=18654.45\ty=13643.92 \nLabel=Strip\t717\tX=18302.35\ty=13702.26 \nLabel=Strip\t718\tX=18649.14\ty=13799.64 \nLabel=Strip\t719\tX=18297.02\ty=13857.84 \nLabel=Strip\t720\tX=18643.78\ty=13955.35 \nLabel=Strip\t721\tX=18291.63\ty=14013.43 \nLabel=Strip\t722\tX=18638.35\ty=14111.07 \nLabel=Strip\t723\tX=18286.19\ty=14169.01 \nLabel=Strip\t724\tX=18632.87\ty=14266.79 \nLabel=Strip\t725\tX=18280.68\ty=14324.59 \nLabel=Strip\t726\tX=18627.32\ty=14422.50 \nLabel=Strip\t727\tX=18275.11\ty=14480.17 \nLabel=Strip\t728\tX=18621.72\ty=14578.22 \nLabel=Strip\t729\tX=18269.48\ty=14635.75 \nLabel=Strip\t730\tX=18616.05\ty=14733.93 \nLabel=Strip\t731\tX=18263.80\ty=14791.32 \nLabel=Strip\t732\tX=18610.33\ty=14889.64 \nLabel=Strip\t733\tX=18258.01\ty=14947.56 \nLabel=Strip\t734\tX=18604.54\ty=15045.35 \nLabel=Strip\t735\tX=18252.24\ty=15102.47 \nLabel=Strip\t736\tX=18598.69\ty=15201.06 \nLabel=Strip\t737\tX=18246.37\ty=15258.05 \nLabel=Strip\t738\tX=18592.79\ty=15356.77 \nLabel=Strip\t739\tX=18240.44\ty=15413.62 \nLabel=Strip\t740\tX=18586.82\ty=15512.48 \nLabel=Strip\t741\tX=18234.45\ty=15569.20 \nLabel=Strip\t742\tX=18580.79\ty=15668.19 \nLabel=Strip\t743\tX=18228.40\ty=15724.77 \nLabel=Strip\t744\tX=18574.70\ty=15823.89 \nLabel=Strip\t745\tX=18222.29\ty=15880.34 \nLabel=Strip\t746\tX=18568.56\ty=15979.60 \nLabel=Strip\t747\tX=18216.12\ty=16035.91 \nLabel=Strip\t748\tX=18562.35\ty=16135.30 \nLabel=Strip\t749\tX=18209.89\ty=16191.48 \nLabel=Strip\t750\tX=18556.08\ty=16291.01 \nLabel=Strip\t751\tX=18203.60\ty=16347.05 \nLabel=Strip\t752\tX=18549.75\ty=16446.71 \nLabel=Strip\t753\tX=18197.25\ty=16502.61 \nLabel=Strip\t754\tX=18543.36\ty=16602.41 \nLabel=Strip\t755\tX=18190.84\ty=16658.18 \nLabel=Strip\t756\tX=18536.91\ty=16758.11 \nLabel=Strip\t757\tX=18184.37\ty=16813.74 \nLabel=Strip\t758\tX=18530.40\ty=16913.81 \nLabel=Strip\t759\tX=18177.84\ty=16969.30 \nLabel=Strip\t760\tX=18523.83\ty=17069.50 \nLabel=Strip\t761\tX=18171.25\ty=17124.87 \nLabel=Strip\t762\tX=18517.20\ty=17225.20 \nLabel=Strip\t763\tX=18164.60\ty=17280.43 \nLabel=Strip\t764\tX=18510.51\ty=17380.89 \nLabel=Strip\t765\tX=18157.89\ty=17435.99 \nLabel=Strip\t766\tX=18503.76\ty=17536.59 \nLabel=Strip\t767\tX=18151.11\ty=17591.54 \nLabel=Strip\t768\tX=18496.95\ty=17692.28 \nLabel=Strip\t769\tX=18144.28\ty=17747.10 \nLabel=Strip\t770\tX=18490.08\ty=17847.97 \nLabel=Strip\t771\tX=18137.39\ty=17902.65 \nLabel=Strip\t772\tX=18483.15\ty=18003.66 \nLabel=Strip\t773\tX=18130.44\ty=18058.21 \nLabel=Strip\t774\tX=18476.16\ty=18159.35 \nLabel=Strip\t775\tX=18123.43\ty=18213.76 \nLabel=Strip\t776\tX=18469.11\ty=18315.03 \nLabel=Strip\t777\tX=18116.35\ty=18369.31 \nLabel=Strip\t778\tX=18461.99\ty=18470.72 \nLabel=Strip\t779\tX=18109.22\ty=18524.86 \nLabel=Strip\t780\tX=18454.82\ty=18626.40 \nLabel=Strip\t781\tX=18102.03\ty=18680.41 \nLabel=Strip\t782\tX=18447.59\ty=18782.08 \nLabel=Strip\t783\tX=18094.77\ty=18835.96 \nLabel=Strip\t784\tX=18440.30\ty=18937.76 \nLabel=Strip\t785\tX=18087.46\ty=18991.50 \nLabel=Strip\t786\tX=18432.94\ty=19093.44 \nLabel=Strip\t787\tX=18080.09\ty=19147.04 \nLabel=Strip\t788\tX=18425.53\ty=19249.12 \nLabel=Strip\t789\tX=18072.65\ty=19302.59 \nLabel=Strip\t790\tX=18418.06\ty=19404.80 \nLabel=Strip\t791\tX=18065.16\ty=19458.13 \nLabel=Strip\t792\tX=18410.52\ty=19560.47 \nLabel=Strip\t793\tX=18057.60\ty=19613.66 \nLabel=Strip\t794\tX=18402.93\ty=19716.14 \nLabel=Strip\t795\tX=18049.99\ty=19769.20 \nLabel=Strip\t796\tX=18395.28\ty=19871.82 \nLabel=Strip\t797\tX=18042.31\ty=19924.74 \nLabel=Strip\t798\tX=18387.56\ty=20027.49 \nLabel=Strip\t799\tX=18034.58\ty=20080.27 \nLabel=Strip\t800\tX=18379.79\ty=20183.15 \nLabel=Strip\t801\tX=18026.78\ty=20235.80 \nLabel=Strip\t802\tX=18371.95\ty=20338.82 \nLabel=Strip\t803\tX=18018.93\ty=20391.33 \nLabel=Strip\t804\tX=18364.06\ty=20494.48 \nLabel=Strip\t805\tX=18011.01\ty=20546.86 \nLabel=Strip\t806\tX=18356.10\ty=20650.15 \nLabel=Strip\t807\tX=18003.04\ty=20702.39 \nLabel=Strip\t808\tX=18348.08\ty=20805.81 \nLabel=Strip\t809\tX=17995.00\ty=20857.91 \nLabel=Strip\t810\tX=18340.01\ty=20961.46 \nLabel=Strip\t811\tX=17986.90\ty=21013.44 \nLabel=Strip\t812\tX=18331.87\ty=21117.12 \nLabel=Strip\t813\tX=17978.75\ty=21168.96 \nLabel=Strip\t814\tX=18323.67\ty=21272.78 \nLabel=Strip\t815\tX=17970.53\ty=21324.48 \nLabel=Strip\t816\tX=18315.42\ty=21428.43 \nLabel=Strip\t817\tX=17962.25\ty=21480.00 \nLabel=Strip\t818\tX=18307.10\ty=21584.08 \nLabel=Strip\t819\tX=17953.92\ty=21635.51 \nLabel=Strip\t820\tX=18298.72\ty=21739.73 \nLabel=Strip\t821\tX=17945.52\ty=21791.03 \nLabel=Strip\t822\tX=18290.29\ty=21895.38 \nLabel=Strip\t823\tX=17937.06\ty=21946.54 \nLabel=Strip\t824\tX=18281.79\ty=22051.02 \nLabel=Strip\t825\tX=17928.54\ty=22102.05 \nLabel=Strip\t826\tX=18273.23\ty=22206.67 \nLabel=Strip\t827\tX=17919.96\ty=22257.55 \nLabel=Strip\t828\tX=18264.61\ty=22362.31 \nLabel=Strip\t829\tX=17911.33\ty=22413.06 \nLabel=Strip\t830\tX=18255.93\ty=22517.95 \nLabel=Strip\t831\tX=17902.63\ty=22568.56 \nLabel=Strip\t832\tX=18247.19\ty=22673.59 \nLabel=Strip\t833\tX=17893.87\ty=22724.07 \nLabel=Strip\t834\tX=18238.39\ty=22829.22 \nLabel=Strip\t835\tX=17885.05\ty=22879.57 \nLabel=Strip\t836\tX=18229.53\ty=22984.86 \nLabel=Strip\t837\tX=17876.17\ty=23035.06 \nLabel=Strip\t838\tX=18220.61\ty=23140.49 \nLabel=Strip\t839\tX=17867.23\ty=23190.56 \nLabel=Strip\t840\tX=18211.63\ty=23296.12 \nLabel=Strip\t841\tX=17858.23\ty=23346.05 \nLabel=Strip\t842\tX=18202.59\ty=23451.74 \nLabel=Strip\t843\tX=17849.17\ty=23501.54 \nLabel=Strip\t844\tX=18193.49\ty=23607.37 \nLabel=Strip\t845\tX=17840.05\ty=23657.03 \nLabel=Strip\t846\tX=18184.33\ty=23762.99 \nLabel=Strip\t847\tX=17830.87\ty=23812.52 \nLabel=Strip\t848\tX=18175.11\ty=23918.61 \nLabel=Strip\t849\tX=17821.63\ty=23968.00 \nLabel=Strip\t850\tX=18165.83\ty=24074.23 \nLabel=Strip\t851\tX=17812.33\ty=24123.48 \nLabel=Strip\t852\tX=18156.49\ty=24229.84 \nLabel=Strip\t853\tX=17802.97\ty=24278.96 \nLabel=Strip\t854\tX=18147.08\ty=24385.46 \nLabel=Strip\t855\tX=17793.55\ty=24434.44 \nLabel=Strip\t856\tX=18137.62\ty=24541.07 \nLabel=Strip\t857\tX=17784.07\ty=24589.92 \nLabel=Strip\t858\tX=18128.10\ty=24696.68 \nLabel=Strip\t859\tX=17774.53\ty=24745.39 \nLabel=Strip\t860\tX=18118.52\ty=24852.28 \nLabel=Strip\t861\tX=17764.92\ty=24900.86 \nLabel=Strip\t862\tX=18108.87\ty=25007.89 \nLabel=Strip\t
